vi "Initialize Destination.vi"(8 "Error In":errorcluster, 10 "For":T1(ring)=enum."User", 11 "Destination In":refnum<vi>) -> (0 "Error Out":errorcluster, 2 "Change Made?":bool, 3 "Destination Out":refnum<vi>)   [LabVIEW 2018, in "Tools Menu.lvlib"]
uses:
  Tools Menu.lvlib
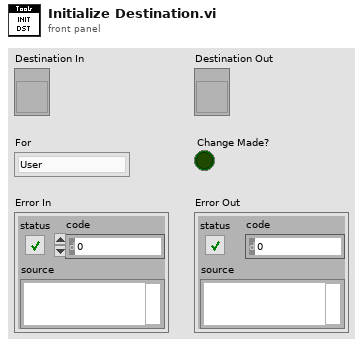
[diagram p1: front panel]
types:
  T1 = enum16{"System", "User", "Project (Visible)", "Project (Hidden)", "Custom..."}
  T2 = enum8{"Enabled", "Disabled", "Disabled and Grayed Out"}
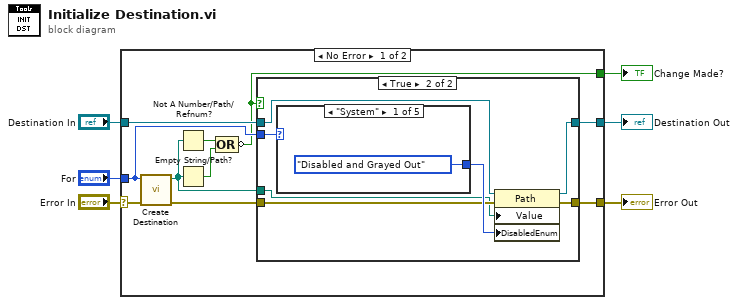
[diagram p0: block diagram]
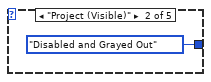
[diagram p3: hidden frame]
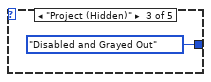
[diagram p4: hidden frame]
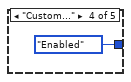
[diagram p5: hidden frame]
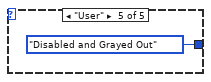
[diagram p6: hidden frame]
diagram:
  n1 = case shown="No Error" "Error In" {
    selector: "Error In" -> [w12 w31]
    tunnel: "For" -> [w9 _]
    tunnel: [w16 w31] -> w5
    tunnel: "Destination In" -> [w14 w32]
    tunnel: [w13 w32] -> w3
    tunnel: [w7 _] -> w1
    frame No Error {
      n2 = call "Create Destination.vi"("Error In"=w12, "For"=w9) -> ("Error Out"=w15:errorcluster, "Destination"=w8:path)  [unwired: 8 in]
      n3 = Not A Number/Path/Refnum?(number/path/refnum=w8) -> (NaN/Path/Refnum?=w10:bool)
      n4 = Empty String/Path?(string/path=w8) -> (empty?=w11:bool)
      n5 = Compound Arithmetic op=OR(w10, w11) -> (invert w7:bool)
      n6 = case shown="True" w7 {
        tunnel: [w17 w24] -> w16
        tunnel: w15 -> [w17 w23]
        tunnel: w14 -> [w18 w22]
        tunnel: [w18 w21] -> w13
        tunnel: w9 -> [_ w20]
        tunnel: w8 -> [_ w19]
        frame False {
        }
        frame True {
          n7 = case shown="\"System\"" w20 {
            tunnel: [T2."Disabled and Grayed Out" ("Disabled") T2."Disabled and Grayed Out" ("Disabled") T2."Disabled and Grayed Out" ("Disabled") T2."Enabled" ("Disabled") T2."Disabled and Grayed Out" ("Disabled")] -> w25
            frame "System" {
            }
            frame "Project (Visible)" {
            }
            frame "Project (Hidden)" {
            }
            frame "Custom..." {
            }
            frame "User" {
            }
          }
          n8 = property on="Property Node" class="Path"(reference=w22, error in=w23, "Value"=w19, "DisabledEnum"=w25) -> (reference out=w21:refnum<vi>, error out=w24:errorcluster)
        }
      }
    }
    frame Error {
    }
  }
  "Error Out" <- w5
  "Destination Out" <- w3
  "Change Made?" <- w1
